vi "Odometry_SwerveKinematics_NewX.vi"(11 "Distances From Center":T1[](array[typedef]) {"Y" format="%14.3f"; "X" format="%14.3f"}) -> (3 "SWERVE_DRIVE_KINEMATICS Out":T2 {"SavedModuleStates"."Angle"."SIN" format="%13.4f"; "SavedModuleStates"."Angle"."COS" format="%13.4f"; "SavedModuleStates"."Angle"."VALUE" format="%13.4f"; "PrevCoR"."Y" format="%14.3f"; "PrevCoR"."X" format="%14.3f"; "Modules"."Y" format="%14.3f"; "Modules"."X" format="%14.3f"})   [LabVIEW 2023, in "Swerve_Odometry_SEN.lvlib"]
doc: "Constructs a swerve drive kinematics object. This takes in a variable number of wheel locations as Translation2ds. The order in which you pass in the wheel locations is the same order that you will recieve the module states when performing inverse kinematics. It is also expected that you pass in the module states in the same order when calling the forward kinematics methods.\n\nThis is a helper class that converts a chassis velocity (dx, dy, and dtheta components) into individual module states (speed and angle).\n \nThe inverse kinematics (converting from a desired chassis velocity to individual module states) uses the relative locations of the modules with respect to the center of rotation. The center of rotation for inverse kinematics is also variable. This means that you can set your set your center of rotation in a corner of the robot to perform special evasion manuevers.\n \nForward kinematics (converting an array of module states into the overall chassis motion) is performs the exact opposite of what inverse kinematics does. Since this is an overdetermined system (more equations than variables), we use a least-squares approximation.\n \nThe inverse kinematics: [moduleStates] = [moduleLocations][chassisSpeeds] We take the Moore-Penrose pseudoinverse of [moduleLocations] and then multiply by [moduleStates] to get our chassis speeds.\n \nForward kinematics is also used for odometry -- determining the position of the robot on the field using encoders and a gyro.\n\nParameters: \n - wheels - Array of Translation data structures indicating the locations of the wheels relative to the physical center of the robot. (Meters)\n\nReturns:\n - SwerveDriveKinematics - The initialized data structure"
uses:
  Swerve_Odometry_SEN.lvlib
  Cluster_SWERVE_DRIVE_KINEMATICS.ctl
  <vilib>/Analysis/Matrix/Datatypes/RealMatrix.ctl
  Cluster_TRANSLATION2D.ctl
  Cluster_SWERVE_DRIVE_MODULE_STATE.ctl
  Cluster_ROTATION2D.ctl
  <vilib>/Analysis/_algsub.llb/Real PseudoInverse Matrix.vi
  Kinimatics_Matrix_CoerceSize.vi
  <vilib>/Analysis/Matrix/NI_Matrix.lvlib
  <vilib>/Analysis/NI_AALPro.lvlib
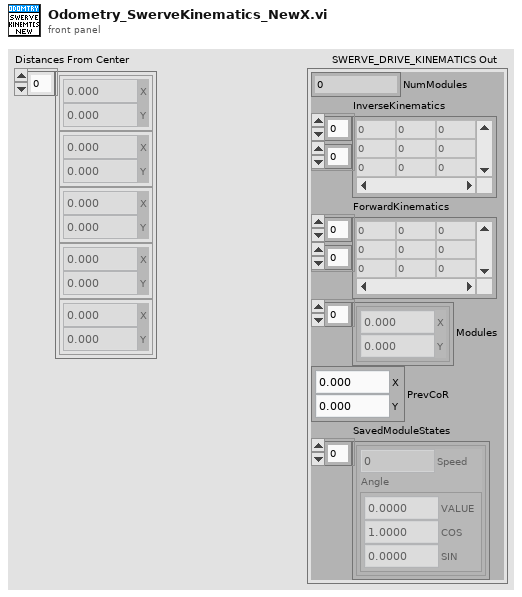
[diagram p1: front panel]
types:
  T1 = typedef "Swerve_Odometry_SEN.lvlib/Cluster_TRANSLATION2D.ctl" = cluster{"X":dbl, "Y":dbl}
  T2 = typedef "Swerve_Odometry_SEN.lvlib/Cluster_SWERVE_DRIVE_KINEMATICS.ctl" = cluster{"NumModules":i32, "InverseKinematics":T3, "ForwardKinematics":T3, "Modules":T1[], "PrevCoR":T1, "SavedModuleStates":T4[]}
  T3 = typedef "NI_Matrix.lvlib/RealMatrix.ctl" = dbl[][]
  T4 = typedef "Swerve_Odometry_SEN.lvlib/Cluster_SWERVE_DRIVE_MODULE_STATE.ctl" = cluster{"Speed":dbl, "Angle":T5}
  T5 = typedef "Swerve_Odometry_SEN.lvlib/Cluster_ROTATION2D.ctl" = cluster{"VALUE":dbl, "COS":dbl, "SIN":dbl}
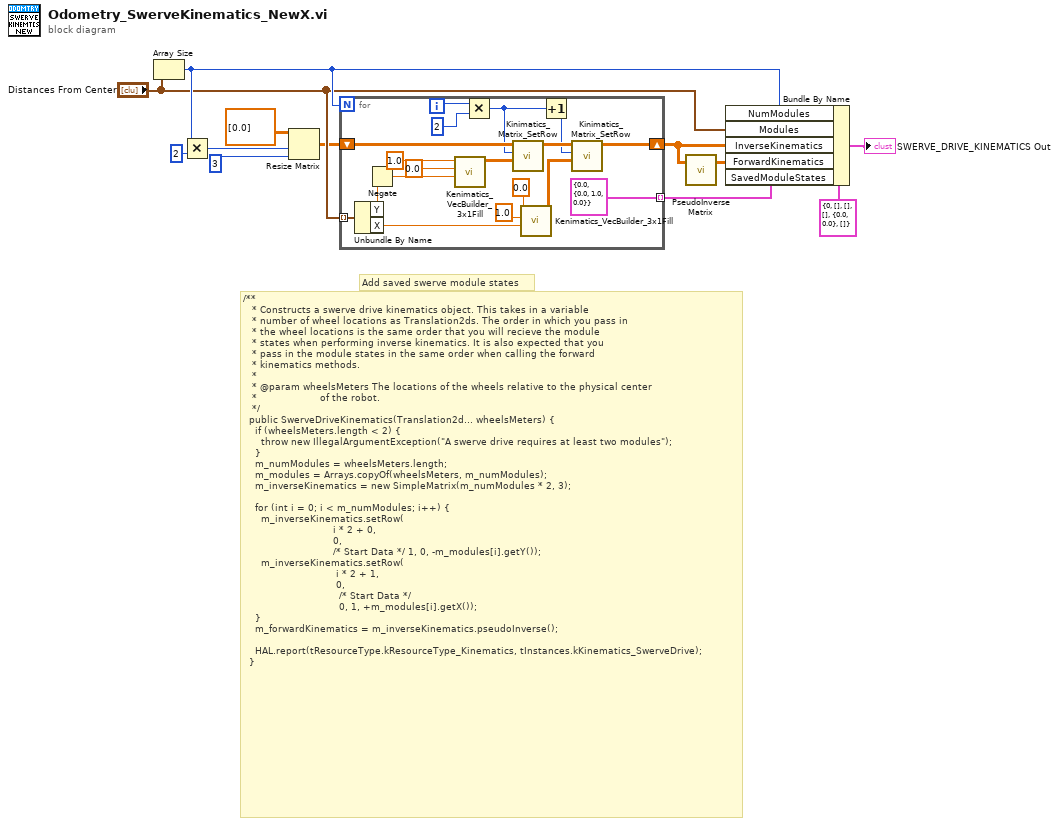
[diagram p0: block diagram]
diagram:
  # "Add saved swerve module states"
  # "/**\n   * Constructs a swerve drive kinematics object. This takes in a variable\n   * number of wheel locations as Translation2ds. The order in which you pass in\n   * the wheel locations is the same order that you will recieve the module\n   * states when performing inverse kinematics. It is also expected that you\n   * pass in the module states in the same order when calling the forward\n   * kinematics methods.\n   *\n   * @param wheelsMeters The locations of the wheels relative to the physical center\n   *                     of the robot.\n   */\n  public SwerveDriveKinematics(Translation2d... wheelsMeters) {\n    if (wheelsMeters.length < 2) {\n      throw new IllegalArgumentException(\"A swerve drive requires at least two modules\");\n    }\n    m_numModules = wheelsMeters.length;\n    m_modules = Arrays.copyOf(wheelsMeters, m_numModules);\n    m_inverseKinematics = new SimpleMatrix(m_numModules * 2, 3);\n\n    for (int i = 0; i < m_numModules; i++) {\n      m_inverseKinematics.setRow(\n                              i * 2 + 0, \n                              0, \n                              /* Start Data */ 1, 0, -m_modules[i].getY());\n      m_inverseKinematics.setRow(\n                               i * 2 + 1, \n                               0, \n                                /* Start Data */ \n                                0, 1, +m_modules[i].getX());\n    }\n    m_forwardKinematics = m_inverseKinematics.pseudoInverse();\n\n    HAL.report(tResourceType.kResourceType_Kinematics, tInstances.kKinematics_SwerveDrive);\n  }"
  n1 = Array Size(array="Distances From Center") -> (size(s)=w8:i32)
  n2 = Multiply(x=w8, y=2) -> (x*y=w2:i32)
  n3 = Resize Matrix(1:3 ("number of columns"), 2:w2, 4:T3 [[0.0]] ("matrix")) -> (0:w1:T3)
  n4 = for {
    N: w8 -> [_]
    shift-right: [w18] -> w6
    shift-left: w1 -> [w20]
    tunnel: "Distances From Center" -> [w28] mode=indexing
    tunnel: [T4 {"Speed"=0.0, "Angle"={"VALUE"=0.0, "COS"=1.0, "SIN"=0.0}} ("SWERVE_DRIVE_MODULE_STATE")] -> w5 mode=indexing
    i -> [w30]
    n5 = Unbundle By Name(w28) -> ("Y"=w27:dbl, "X"=w13:dbl)
    n6 = Negate(x=w27) -> (-x=w15:dbl)
    n7 = call "Kenimatics_VecBuilder_3x1Fill.vi"("R2"=w15, "R1"=0.0, "R0"=1.0) -> ("output matrix"=w25:T3)  [unwired: 8 in]
    n8 = Multiply(x=w30, y=2) -> (x*y=w17:i32)
    n9 = call "Kinimatics_Matrix_SetRow.vi"("Fill Row Vector"=w25, "Row"=w17, "input matrix"=w20) -> ("output matrix"=w19:T3)  [unwired: 7 in, 1 out]
    n10 = call "Kenimatics_VecBuilder_3x1Fill.vi"("R2"=w13, "R1"=1.0, "R0"=0.0) -> ("output matrix"=w26:T3)  [unwired: 8 in]
    n11 = Increment(x=w17) -> (x+1=w16:i32)
    n12 = call "Kinimatics_Matrix_SetRow.vi"("Fill Row Vector"=w26, "Row"=w16, "input matrix"=w19) -> ("output matrix"=w18:T3)  [unwired: 7 in, 1 out]
  }
  n13 = call-poly <vilib>:"PseudoInverse Matrix.vi"("Input Matrix"=w6) -> ("PseudoInverse Matrix"=w9:T3)  [unwired: 1 in, 1 out]
  n14 = Bundle By Name(cluster=T2 {"NumModules"=0, "InverseKinematics"=[], "ForwardKinematics"=[], "Modules"=[], "PrevCoR"={"X"=0.0, "Y"=0.0}, "SavedModuleStates"=[]} ("SWERVE_DRIVE_KINEMATICS"), "NumModules"=w8, "Modules"="Distances From Center", "InverseKinematics"=w6, "ForwardKinematics"=w9, "SavedModuleStates"=w5) -> (→"SWERVE_DRIVE_KINEMATICS Out":T2)
